vi "Construct Page Map.vi"(8 "error in (no error)":errorcluster, 10 "Top Page ID":string, 11 "Confluence Connection in":refnum<class "Confluence.lvclass">) -> (0 "error out":errorcluster, 1 "Top Page Title":string, 2 "Page Map":map{string, T1}(c390), 3 "Confluence out":refnum<class "Confluence.lvclass">)   [LabVIEW 2023, in "VIDoc Printer - Confluence.lvlib" / "VIDoc Printer - Confluence.lvclass"]
uses:
  VIDoc Printer - Confluence.lvclass
  <userlib>/_PetranWay/LabVIEW Confluence API/Source/Confluence/Confluence Connection/Confluence.lvclass
  Types/Page Info.ctl
  <userlib>/_PetranWay/LabVIEW Confluence API/Source/Confluence/Page/Page.lvclass
  <userlib>/_PetranWay/LabVIEW Confluence API/Source/Confluence/Page/Page.lvclass/Page.ctl
  <userlib>/_PetranWay/LabVIEW Confluence API/Source/Confluence/Page/Accessors/Read title.vi
  <userlib>/_PetranWay/LabVIEW Confluence API/Source/Confluence/Page/Accessors/Read storage value.vi
  <vilib>/JDP Science/JSONtext/Find Item.vi
  <userlib>/_PetranWay/LabVIEW Atlassian API/Source/JSON Utilities/Strip Quotes Around String.vi
  <userlib>/_PetranWay/LabVIEW Confluence API/Source/Confluence/Page/Accessors/Read storage value.vi/24cc900c-cd5f-46ff-be78-0781b543e64e.vi
  <vilib>/JDP Science/JSONtext/Next JSON Value.vi
  <vilib>/JDP Science/JSONtext/String Subset.vi
  <vilib>/JDP Science/JSONtext/Parsing/Advance past next JSON Value (inlined COPY).vi
  <vilib>/JDP Science/JSONtext/Parsing/Advance past whitespace.vi
  <vilib>/JDP Science/JSONtext/Parsing/Advance past String.vi
  <vilib>/JDP Science/JSONtext/Parsing/Advance past Number.vi
  <vilib>/JDP Science/JSONtext/Parsing/Advance past Line Ending.vi
  <vilib>/JDP Science/JSONtext/Parsing/Parse Full Path or Item Name.vi
  <vilib>/JDP Science/JSONtext/Parsing/Advance past Array.vi
  <vilib>/JDP Science/JSONtext/Parsing/Advance past Object.vi
  <vilib>/JDP Science/JSONtext/support/Error Cluster From Code.vi
  <vilib>/JDP Science/JSONtext/Offset/Find Item Locations by Path.vi
  <vilib>/JDP Science/JSONtext/JSON text to Variant.vi
  <vilib>/JDP Science/JSONtext/LVClass Serializer/JSONtext LVClass Serializer.lvclass
  <userlib>/_PetranWay/LabVIEW Confluence API/Source/Confluence/iConfluence/iConfluence.lvclass
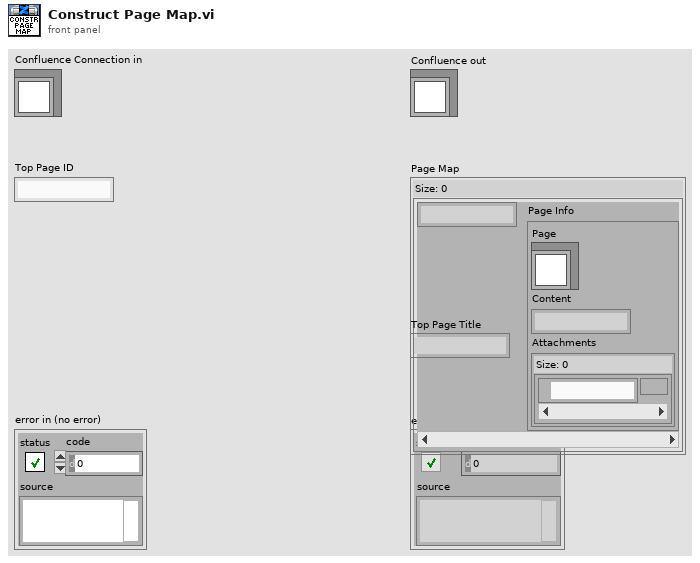
[diagram p1: front panel]
types:
  T1 = typedef "VIDoc Printer - Confluence.lvlib/VIDoc Printer - Confluence.lvclass/Page Info.ctl" = cluster{"Page":refnum<class "Page.lvclass">, "Content":string, "Attachments":set{path}}
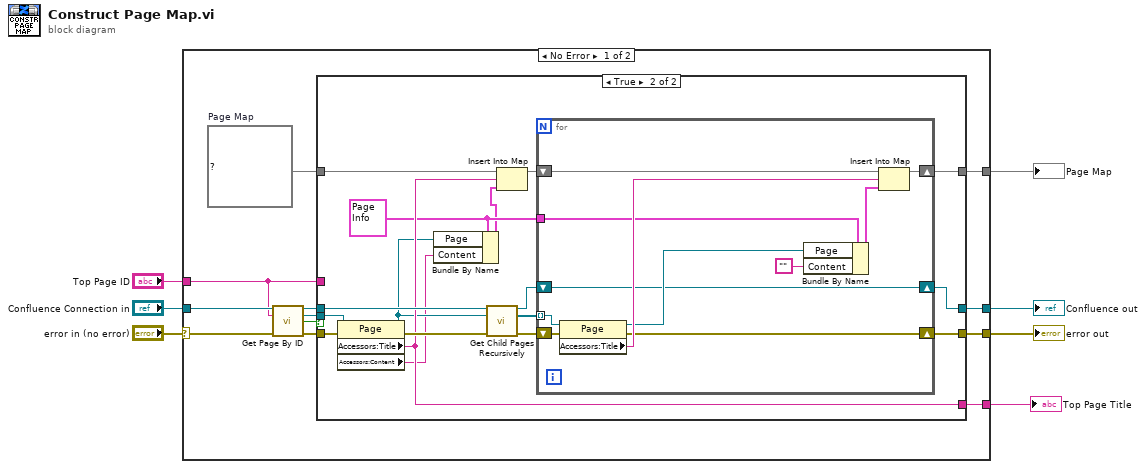
[diagram p0: block diagram]
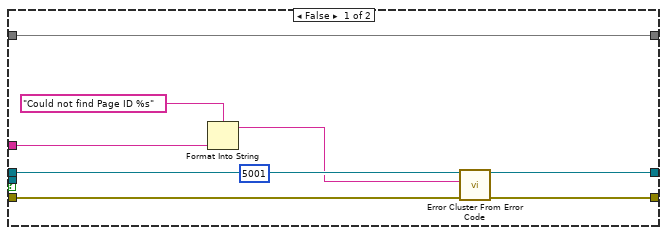
[diagram p2: hidden frame]
diagram:
  n1 = case shown="No Error" "error in (no error)" {
    selector: "error in (no error)" -> [w18 w57]
    tunnel: "Confluence Connection in" -> [w19 w56]
    tunnel: [w12 w56] -> w5
    tunnel: [w11 w57] -> w4
    tunnel: "Top Page ID" -> [w10 _]
    tunnel: [w9 _] -> w2
    tunnel: [w8 _] -> w1
    frame No Error {
      w16 = map{string, T1} {}  # Page Map
      n2 = call-dynamic "Get Page By ID.vi"("Confluence Connection in"=w19, "ID"=w10, "error in (no error)"=w18) -> ("Atlassian Connection out"=w13:refnum<class "Confluence.lvclass">, "Page out"=w17:refnum<class "Page.lvclass">, "Found"=w14:bool, "error out"=w15:errorcluster)  [unwired: 9 in]
      n3 = case shown="True" w14 {
        tunnel: w17 -> [_ w44]
        tunnel: w16 -> [w20 w43]
        tunnel: w15 -> [w24 w42]
        tunnel: w13 -> [w27 w40]
        tunnel: [w27 w28] -> w12
        tunnel: [w25 w36] -> w11
        tunnel: w10 -> [w22 _]
        tunnel: [w20 w35] -> w9
        tunnel: [_ w34] -> w8
        frame False {
          n4 = Format Into String(format string="Could not find Page ID %s", w22) -> (resulting string=w21:string)  [unwired: 2 in, 1 out]
          n5 = call <vilib>:"Error Cluster From Error Code.vi"("error in (no error)"=w24, "error message (\"\")"=w21, "error code (0)"=5001) -> ("error out"=w25:errorcluster)  [unwired: 6 in]
        }
        frame True {
          w33 = T1 {"Page"=refnum, "Content"="", "Attachments"={}} ("Page Info")
          n6 = property class="Page"(reference=w44, error in=w42) -> (reference out=w32:refnum<class "Page.lvclass">, error out=w41:errorcluster, "Accessors:Title"=w34:string, "Accessors:Content"=w31:string)
          n7 = Bundle By Name(cluster=w33, "Page"=w32, "Content"=w31) -> (w30:T1)
          n8 = call-dynamic "Get Child Pages Recursively.vi"("Confluence in"=w40, "Page"=w32, "error in (no error)"=w41) -> ("Confluence out"=w29:refnum<class "Confluence.lvclass">, "Child Pages"=w38:refnum<class "Page.lvclass">[], "error out"=w37:errorcluster)  [unwired: 9 in, 1 out]
          n9 = Insert Into Map(map in=w43, key=w34, value=w30) -> (map out=w39:map{string, T1})  [unwired: 2 out]
          n10 = for {
            shift-right: [w51] -> w35
            shift-left: w39 -> [w55]
            tunnel: w38 -> [w54] mode=indexing
            shift-right: [w50] -> w36
            shift-left: w37 -> [w53]
            tunnel: w33 -> [w47]
            shift-right: [w46] -> w28
            shift-left: w29 -> [w46]
            n11 = property class="Page"(reference=w54, error in=w53) -> (reference out=w49:refnum<class "Page.lvclass">, error out=w50:errorcluster, "Accessors:Title"=w52:string)
            n12 = Bundle By Name(cluster=w47, "Page"=w49, "Content"="") -> (w48:T1)
            n13 = Insert Into Map(map in=w55, key=w52, value=w48) -> (map out=w51:map{string, T1})  [unwired: 2 out]
          }
        }
      }
    }
    frame Error {
    }
  }
  "Confluence out" <- w5
  "error out" <- w4
  "Page Map" <- w2
  "Top Page Title" <- w1
